vi "Open.vi"(8 "error in (no error)":errorcluster, 10 "Link":cluster{"IP":string, "Port":u16}, 11 "PEU in":refnum<class "PEU.lvclass">) -> (0 "error out":errorcluster, 2 "Link_OK":bool, 3 "PEU out":refnum<class "PEU.lvclass">)   [LabVIEW 2020, in "PEU.lvlib" / "PEU.lvclass"]
uses:
  PEU.lvclass
  PEU.lvclass/PEU.ctl
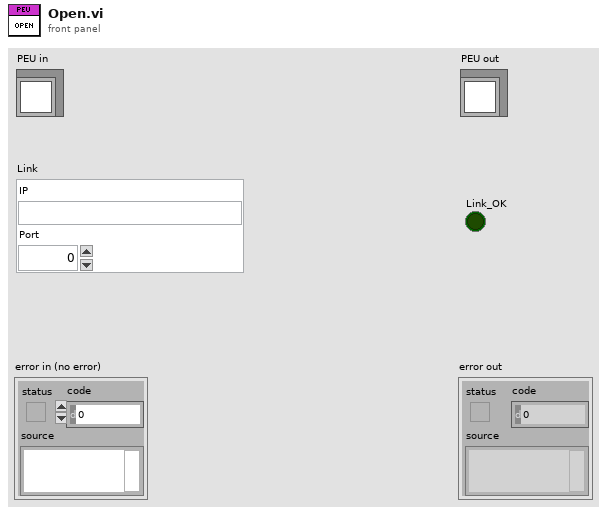
[diagram p1: front panel]
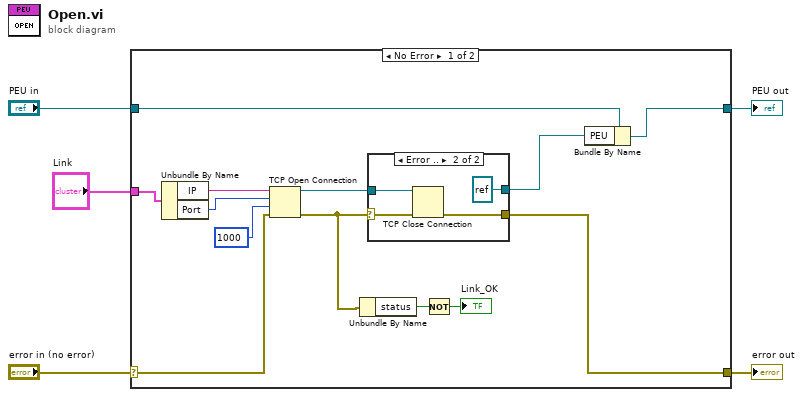
[diagram p0: block diagram]
diagram:
  n1 = case shown="No Error" "error in (no error)" {
    selector: "error in (no error)" -> [w13 w26]
    tunnel: [w7 w26] -> w4
    tunnel: [w14 w25] -> w2
    tunnel: "PEU in" -> [w15 w25]
    tunnel: "Link" -> [w18 _]
    frame No Error {
      n2 = Unbundle By Name(w18) -> ("IP"=w17:string, "Port"=w16:u16)
      n3 = TCP Open Connection(address=w17, remote port or service name=w16, timeout ms (60000)=1000, error in (no error)=w13) -> (connection ID=w12:refnum<k5>, error out=w8:errorcluster)  [unwired: 1 in]
      n4 = Unbundle By Name(w8) -> ("status"=w10:bool)
      n5 = case shown="Error .." w8 {
        selector: w8 -> [w19 w24]
        tunnel: w12 -> [w20 w23]
        tunnel: [w20 refnum<k5> refnum ("connection ID")] -> w11
        tunnel: [w19 w21] -> w7
        frame No Error {
        }
        frame Error {
          n6 = TCP Close Connection(connection ID=w23, error in (no error)=w24) -> (error out=w21:errorcluster)  [unwired: 1 in, 1 out]
        }
      }
      n7 = Not(x=w10) -> (.not. x?=→"Link_OK":bool)
      n8 = Bundle By Name(cluster=w15, "PEU"=w11) -> (w14:refnum<class "PEU.lvclass">)
    }
    frame Error {
    }
  }
  "error out" <- w4
  "PEU out" <- w2
